vi "LM3Sxxxx_Interrupt_Template.vi"(10 "param":u32, 11 "vector":T1(ring)=enum."Timer 1") -> ()   [LabVIEW 2011]
doc: "Interrupt template for LabVIEW Embedded targets. This handler VI can be used to handle all interrupts (or it can be duplicated for each interrupt)."
panel:
  # "This VI will run as an interrupt service routine."
  # "vector indentifies the interrupt vector number for the interrupt."
  # "param contains the current value of the interrupt status register. Use param to determine the source of the interrupt.  For example, when a GPIO interrupt occurs, use this value to determine which pin triggered the interrupt."
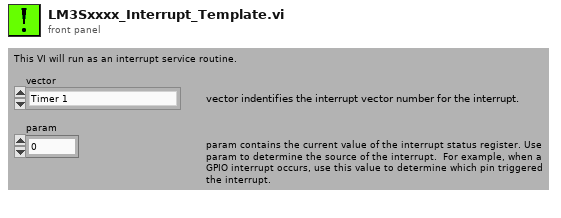
[diagram p1: front panel]
types:
  T1 = enum32{"Unused 0", "Unused 1", "Unused 2", "Unused 3", "Unused 4", "Unused 5", "Unused 6", "Unused 7", "Unused 8", "Unused 9", "Unused 10", "Unused 11", "Unused 12", "Unused 13", "Unused 14", "Unused 15", "GPIO A", "GPIO B", "GPIO C", "GPIO D", "GPIO E", "Unused 21", "Unused 22", "Unused 23", "Unused 24", "PWM Fault", "PWM Generator 0", "PWM Generator 1", "PWM Generator 2", "QEI 0", "ADC Sequence 0", "ADC Sequence 1", "ADC Sequence 2", "Unused 33", "Watchdog Timer", "Timer 0", "Unused 36", "Timer 1", "Unused 38", "Timer 2", "Unused 40", "Analog Comparator", "Unused 42", "Unused 43", "Brownout Detection", "Unused 45", "GPIO F", "GPIO G", "Unused 48", "Unused 49", "Unused 50", "Timer 3", "Unused 52", "Unused 53", "QEI 1"}
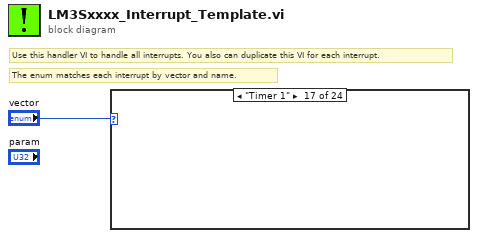
[diagram p0: block diagram]
diagram:
  # "The enum matches each interrupt by vector and name."
  # "Use this handler VI to handle all interrupts. You also can duplicate this VI for each interrupt."
  n1 = case shown="\"Timer 1\"" "vector" {
    frame Default {
      # "Unknown / unexpected interrupt"
    }
    frame "GPIO A" {
    }
    frame "GPIO B" {
    }
    frame "GPIO C" {
    }
    frame "GPIO D" {
    }
    frame "GPIO E" {
    }
    frame "PWM Fault" {
    }
    frame "PWM Generator 0" {
    }
    frame "PWM Generator 1" {
    }
    frame "PWM Generator 2" {
    }
    frame "QEI 0" {
    }
    frame "ADC Sequence 0" {
    }
    frame "ADC Sequence 1" {
    }
    frame "ADC Sequence 2" {
    }
    frame "Watchdog Timer" {
    }
    frame "Timer 0" {
    }
    frame "Timer 1" {
    }
    frame "Timer 2" {
    }
    frame "Analog Comparator" {
    }
    frame "Brownout Detection" {
    }
    frame "GPIO F" {
    }
    frame "GPIO G" {
    }
    frame "Timer 3" {
    }
    frame "QEI 1" {
    }
  }
